vi "Set Language (SubVI).vi"(6 "Language (English)":enum16{"English", "Deutsch", "Italiano"}(ring), 7 "Simulation \nReferences":T3, 8 "error in (no error)":errorcluster, 9 "Status\nReferences":T1, 10 "Selection \nReferences":T2, 11 "Language Data":string[][](array[string])) -> (0 "error out":errorcluster, 3 "Language Data Out":string[][](array[string]))   [LabVIEW 2017]
panel:
  # "input values"
  # "references"
  # "output values"
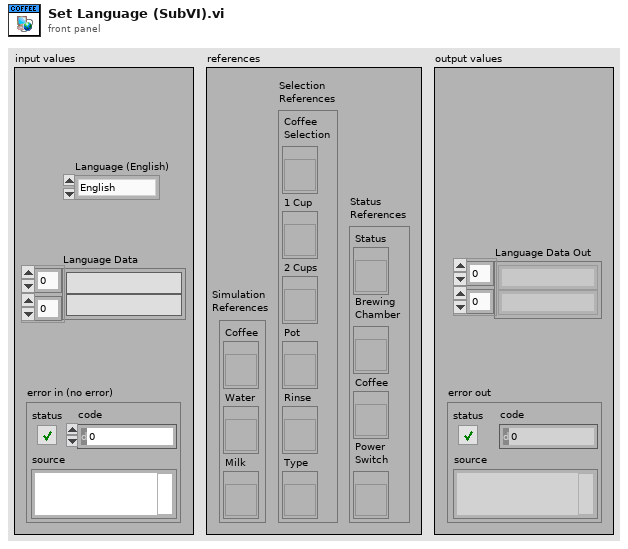
[diagram p1: front panel]
types:
  T1 = cluster{"Status":refnum<vi>, "Brewing \nChamber":refnum<vi>, "Coffee":refnum<vi>, "Power \nSwitch":refnum<vi>}
  T2 = cluster{"Coffee \nSelection":refnum<vi>, "1 Cup":refnum<vi>, "2 Cups":refnum<vi>, "Pot":refnum<vi>, "Rinse":refnum<vi>, "Type":refnum<vi>}
  T3 = cluster{"Coffee":refnum<vi>, "Water":refnum<vi>, "Milk":refnum<vi>}
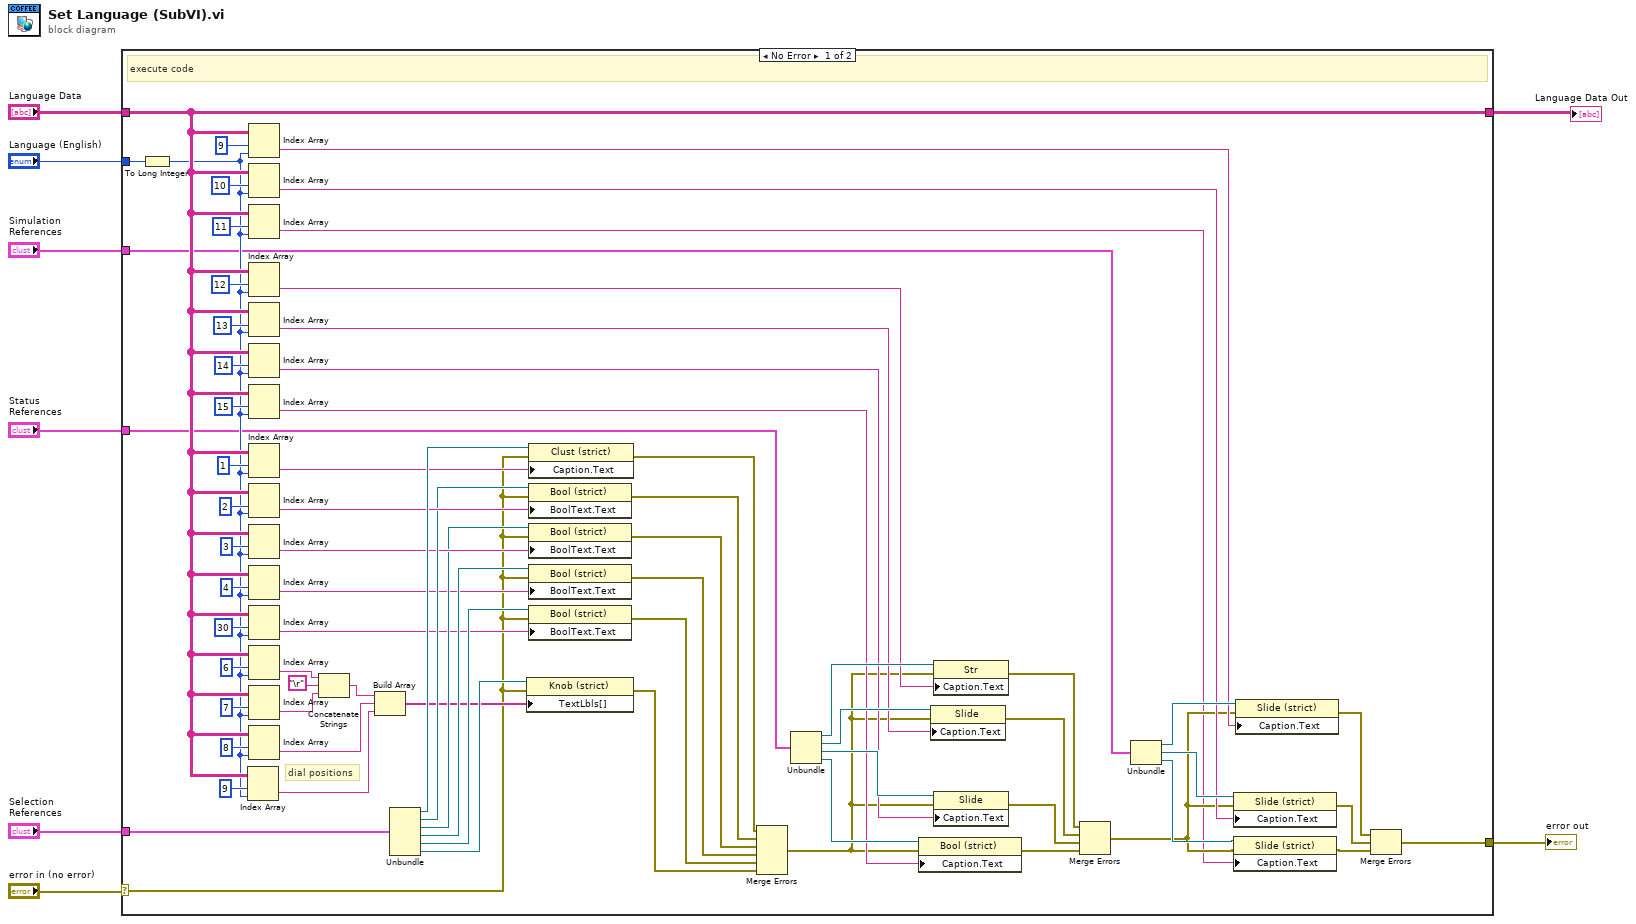
[diagram p0: block diagram]
diagram:
  n1 = case shown="No Error" "error in (no error)" {
    selector: "error in (no error)" -> [w39 w81]
    tunnel: [w9 w81] -> w7
    tunnel: "Simulation \nReferences" -> [w11 _]
    tunnel: "Language Data" -> [w28 w80]
    tunnel: [w28 w80] -> w4
    tunnel: "Language (English)" -> [w76 _]
    tunnel: "Status\nReferences" -> [w12 _]
    tunnel: "Selection \nReferences" -> [w10 _]
    frame No Error {
      # "dial positions"
      # "execute code"
      n2 = To Long Integer(number=w76) -> (32bit integer=w27:i32)
      n3 = Index Array(array=w28, index (row)=9 ("disabled index (row)"), index (col)=w27) -> (element=w29:string)
      n4 = Index Array(array=w28, index (row)=9 ("disabled index (row)"), index (col)=w27) -> (element=w21:string)
      n5 = Index Array(array=w28, index (row)=10 ("index (col)"), index (col)=w27) -> (element=w18:string)
      n6 = Index Array(array=w28, index (row)=11 ("disabled index (row)"), index (col)=w27) -> (element=w14:string)
      n7 = Index Array(array=w28, index (row)=12 ("disabled index (row)"), index (col)=w27) -> (element=w63:string)
      n8 = Index Array(array=w28, index (row)=13 ("index (col)"), index (col)=w27) -> (element=w62:string)
      n9 = Index Array(array=w28, index (row)=14 ("disabled index (row)"), index (col)=w27) -> (element=w61:string)
      n10 = Index Array(array=w28, index (row)=15 ("disabled index (row)"), index (col)=w27) -> (element=w60:string)
      n11 = Index Array(array=w28, index (row)=1 ("disabled index (row)"), index (col)=w27) -> (element=w50:string)
      n12 = Index Array(array=w28, index (row)=2 ("index (col)"), index (col)=w27) -> (element=w49:string)
      n13 = Index Array(array=w28, index (row)=3 ("disabled index (row)"), index (col)=w27) -> (element=w47:string)
      n14 = Index Array(array=w28, index (row)=4 ("disabled index (row)"), index (col)=w27) -> (element=w44:string)
      n15 = Index Array(array=w28, index (row)=30 ("disabled index (row)"), index (col)=w27) -> (element=w42:string)
      n16 = Index Array(array=w28, index (row)=6 ("disabled index (row)"), index (col)=w27) -> (element=w25:string)
      n17 = Index Array(array=w28, index (row)=7 ("disabled index (row)"), index (col)=w27) -> (element=w24:string)
      n18 = Index Array(array=w28, index (row)=8 ("disabled index (row)"), index (col)=w27) -> (element=w26:string)
      n19 = Concatenate Strings(w25, "\r", w24) -> (w23:string)
      n20 = Build Array(w23, w26, w29) -> (w40:string[])
      n21 = Unbundle(w10) -> ("Coffee \nSelection"=w51:refnum<vi>, "1 Cup"=w48:refnum<vi>, "2 Cups"=w46:refnum<vi>, "Pot"=w45:refnum<vi>, "Rinse"=w43:refnum<vi>, "Type"=w41:refnum<vi>)
      n22 = property class="Knob (strict)"(reference=w41, error in=w39, "TextLbls[]"=w40) -> (error out=w33:errorcluster)  [unwired: 1 out]
      n23 = property class="Clust (strict)"(reference=w51, error in=w39, "Caption.Text"=w50) -> (error out=w38:errorcluster)  [unwired: 1 out]
      n24 = property class="Bool (strict)"(reference=w48, error in=w39, "BoolText.Text"=w49) -> (error out=w37:errorcluster)  [unwired: 1 out]
      n25 = property class="Bool (strict)"(reference=w46, error in=w39, "BoolText.Text"=w47) -> (error out=w36:errorcluster)  [unwired: 1 out]
      n26 = property class="Bool (strict)"(reference=w45, error in=w39, "BoolText.Text"=w44) -> (error out=w35:errorcluster)  [unwired: 1 out]
      n27 = property class="Bool (strict)"(reference=w43, error in=w39, "BoolText.Text"=w42) -> (error out=w34:errorcluster)  [unwired: 1 out]
      n28 = Merge Errors(w38, w37, w36, w35, w34, w33) -> (w32:errorcluster)
      n29 = Unbundle(w12) -> ("Status"=w72:refnum<vi>, "Brewing \nChamber"=w71:refnum<vi>, "Coffee"=w70:refnum<vi>, "Power \nSwitch"=w69:refnum<vi>)
      n30 = property class="Bool (strict)"(reference=w69, error in=w32, "Caption.Text"=w60) -> (error out=w64:errorcluster)  [unwired: 1 out]
      n31 = property class="Slide"(reference=w71, error in=w32, "Caption.Text"=w62) -> (error out=w66:errorcluster)  [unwired: 1 out]
      n32 = property class="Str"(reference=w72, error in=w32, "Caption.Text"=w63) -> (error out=w67:errorcluster)  [unwired: 1 out]
      n33 = property class="Slide"(reference=w70, error in=w32, "Caption.Text"=w61) -> (error out=w65:errorcluster)  [unwired: 1 out]
      n34 = Merge Errors(w67, w66, w65, w64) -> (w15:errorcluster)
      n35 = Unbundle(w11) -> ("Coffee"=w22:refnum<vi>, "Water"=w19:refnum<vi>, "Milk"=w16:refnum<vi>)
      n36 = property on="Property Node" class="Slide (strict)"(reference=w19, error in=w15, "Caption.Text"=w18) -> (error out=w17:errorcluster)  [unwired: 1 out]
      n37 = property on="Property Node" class="Slide (strict)"(reference=w16, error in=w15, "Caption.Text"=w14) -> (error out=w13:errorcluster)  [unwired: 1 out]
      n38 = property on="Property Node" class="Slide (strict)"(reference=w22, error in=w15, "Caption.Text"=w21) -> (error out=w20:errorcluster)  [unwired: 1 out]
      n39 = Merge Errors(w20, w17, w13) -> (w9:errorcluster)
    }
    frame Error {
      # "do nothing"
    }
  }
  "error out" <- w7
  "Language Data Out" <- w4
